vi "QMH_Tester_rev1.vi"() -> ()   [LabVIEW 2024]
doc: "Demonstrates the fundamentals of the Queued Message Handler design pattern in LabVIEW. A queued message handler, in its simplest form, is composed of two loops. The Event Handling Loop responds to user interface events by enqueuing \"messages\" on a message queue. These messages are dequeued in the Message Handling Loop. Note that the Message Handling Loop is also capable of sending messages to itself."
uses:
  Controls/Control_Stop.ctl
  Controls/Control_Unitherm Connect Disconnect Bool.ctl
  Controls/Control_M4X Connect Disconnect Bool.ctl
  Controls/Control_Fornax Connect Disconnect Bool.ctl
  Controls/Control_Unitherm Set Load Numeric.ctl
  Controls/Control_Unitherm Set Load Bool.ctl
  Controls/Control_Unitherm VISA Resource.ctl
  Controls/Control_Unitherm Clear Load Bool.ctl
  Controls/Control_PXI-7854R Connect Disconnect Bool.ctl
  Controls/Control_PXI-7854R 75kHz Bool.ctl
  Controls/Control_PXI-7854R uSec Off Numeric.ctl
  Controls/Control_PXI-7854R uSec On Numeric.ctl
  Controls/Control_PXI-7854R Resource.ctl
  Controls/Control_PXI-7854R Set Config Bool.ctl
  Controls/Control_PXI-7854R Set Config Enum.ctl
  Controls/Control_M4X Read Current Bool.ctl
  Controls/Control_Fornax Set Monopolar Command - Energy Channel ID Enum.ctl
  Controls/Control_Fornax Set Monopolar Command Bool.ctl
  Controls/Control_Fornax Set Monopolar Command - Cut Mode Enum.ctl
  Controls/Control_Fornax Set Monopolar Command - Coag Mode Enum.ctl
  Controls/Control_Fornax Set Monopolar Command - Cut Power Command Enum.ctl
  Controls/Control_Fornax Set Monopolar Command - Coag Power Command Enum.ctl
  Controls/Control_Fornax Set Monopolar Command - Serial Number String.ctl
  Program Files/National Instruments/LabVIEW 2024/examples/Design Patterns/Queued Message Handler/support/QMH Fundamentals - Message Cluster.ctl
  Controls/Control_Message Handling Cluster.ctl
  Controls/Control_M4X Connection.ctl
  Controls/Control_PXI-7854R FPGA Reference.ctl
  Controls/Control_Unitherm Connect Disconnect Cluster.ctl
  Controls/Control_PXI-7854R Connect Disconnect Cluster.ctl
  Controls/Control_Fornax Set Monopolar Command Cluster.ctl
  Controls/Control_PXI-7854R Set Config Cluster.ctl
  <vilib>/Utility/error.llb/Error Cluster From Error Code.vi
  <vilib>/rvi/errors/niLvFpgaAdjustHostInterfaceError.vi
  <vilib>/rvi/interface/nirviReadWriteControl/nirviReadWriteControl.xnode
  <vilib>/ErrorRing/Error Ring.xnode
  NiFpgaLv.dll
  <vilib>/rvi/interface/Simulation/niFpgaSimulationCallBeginRW.vi
  <vilib>/rvi/interface/nirviCloseFPGA/nirviCloseFPGA.xnode
  <vilib>/FPGAPlugInAG/Dynamic/niLvFpga_Close_Dynamic.vi
  <vilib>/userDefined/High Color/nirio_resource_hc.ctl
panel:
  in  "Serial Number":T1="T5G00443DX"
  in  "CoagPowerCommand":T2
  in  "CutPowerCommand":T3
  in  "CoagMode":T4
  in  "CutMode":T5
  in  "Fornax Set Monopolar Command":T6
  in  "EnergyChannelID":T7
  out "Data":waveform(dbl)[](graph)
  out "Array":T8(array[cluster])
  in  "Read Current":T9
  in  "7854 Config Enum":T10=enum."Off"
  in  "7854 Set Config":T11
  in  "resource name":T12="PXI1Slot6" caption="RIO Device"
  in  "uSec On":T13=7
  in  "uSec Off":T14=6
  in  "75kHz":T15=TRUE
  in  "7854 Connect/Disconnect":T16
  out "PXI-7854R Connected?":bool
  in  "Clear Load":T17
  in  "Unitherm Refnum in":T18="COM4"
  in  "Set Load":T19
  in  "Load (Ohms)":T20
  out "M4X Connected?":bool
  in  "Fornax Connect/Disconnect":T21
  in  "M4X Connect/Disconnect":T22
  in  "Unitherm Connect/Disconnect":T23
  out "Unitherm Connected?":bool
  out "Fornax Connected?":bool
  out "Display Message":string="\"Stop\" button pressed"
  in  "Fornax Action 1":bool
  in  "Stop":T24
  # "Unitherm"
  # "PXI-7854R"
  # "Fornax"
  # "M4X"
  # "Set Monopolar Command"
  # "Note: If you are creating a LabVIEW application based on the Queued Message Handler design pattern, create a Queued Message Handler project from the File > Create Project dialog."
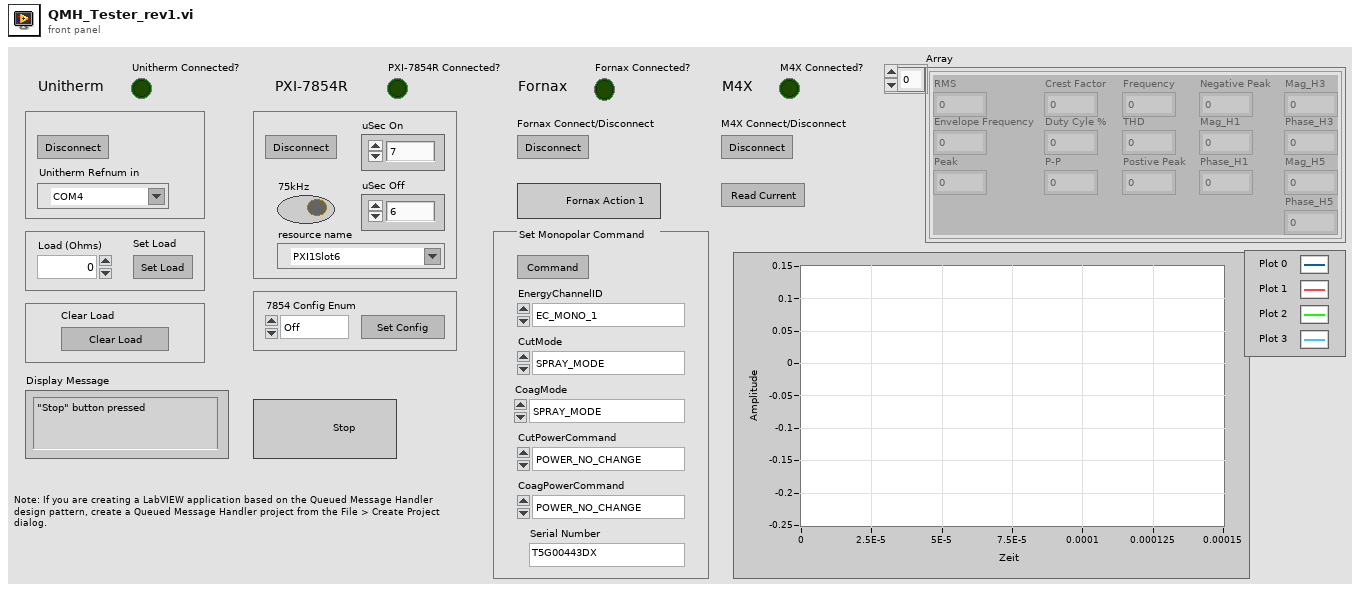
[diagram p1: front panel]
types:
  T1 = typedef "Control_Fornax Set Monopolar Command - Serial Number String.ctl" = string
  T2 = typedef "Control_Fornax Set Monopolar Command - Coag Power Command Enum.ctl" = enum16{"POWER_NO_CHANGE", "POWER_INCREASE", "POWER_DECREASE", "POWER_INCREASE_REPEAT", "POWER_DECREASE_REPEAT"}
  T3 = typedef "Control_Fornax Set Monopolar Command - Cut Power Command Enum.ctl" = enum16{"POWER_NO_CHANGE", "POWER_INCREASE", "POWER_DECREASE", "POWER_INCREASE_REPEAT", "POWER_DECREASE_REPEAT"}
  T4 = typedef "Control_Fornax Set Monopolar Command - Coag Mode Enum.ctl" = enum16{"SPRAY_MODE", "CUT_MODE", "BLEND_MODE", "FULGERATE_MODE", "BEPOLAR_MODE", "VESSEL_SEALING_MODE", "VALLEYLAB_MODE", "BIPOLAR_RESECTION_CUT_MODE", "BIPOLAR_RESECTION_COAG_MODE", "AUTOBIPOLAR_MODE", "VIPER_HLA", "SOFT_COAG_MODE", "NUM_ENERGY_MODES"}
  T5 = typedef "Control_Fornax Set Monopolar Command - Cut Mode Enum.ctl" = enum16{"SPRAY_MODE", "CUT_MODE", "BLEND_MODE", "FULGERATE_MODE", "BIPOLAR_MODE", "VESSEL_SEALING_MODE", "VALLEYLAB_MODE", "BIPOLAR_RESECTION_CUT_MODE", "BIPOLAR_RESECTION_COAG_MODE", "AUTOBIPOLAR_MODE", "VIPER_HLA", "SOFT_COAG_MODE", "NUM_ENERGY_MODES"}
  T6 = typedef "Control_Fornax Set Monopolar Command Bool.ctl" = bool
  T7 = typedef "Control_Fornax Set Monopolar Command - Energy Channel ID Enum.ctl" = enum16{"EC_MONO_1", "EC_BIPOLAR", "EC_MONO_2", "EC_ADVANCED", "NUM_ENERGY_CHANNELS", "EC_NOT_USED"}
  T8 = cluster{"RMS":dbl, "Envelope Frequency":dbl, "Peak":dbl, "Crest Factor":dbl, "Duty Cyle %":dbl, "P-P":dbl, "Frequency":dbl, "THD":dbl, "Postive Peak":dbl, "Negative Peak":dbl, "Mag_H1":dbl, "Phase_H1":dbl, "Mag_H3":dbl, "Phase_H3":dbl, "Mag_H5":dbl, "Phase_H5":dbl}[]
  T9 = typedef "Control_M4X Read Current Bool.ctl" = bool
  T10 = typedef "Control_PXI-7854R Set Config Enum.ctl" = enum16{"Mono 1", "Mono 2", "BiPolar", "LigaSure", "Off"}
  T11 = typedef "Control_PXI-7854R Set Config Bool.ctl" = bool
  T12 = typedef "Control_PXI-7854R Resource.ctl" = tag
  T13 = typedef "Control_PXI-7854R uSec On Numeric.ctl" = u16
  T14 = typedef "Control_PXI-7854R uSec Off Numeric.ctl" = u16
  T15 = typedef "Control_PXI-7854R 75kHz Bool.ctl" = bool
  T16 = typedef "Control_PXI-7854R Connect Disconnect Bool.ctl" = bool
  T17 = typedef "Control_Unitherm Clear Load Bool.ctl" = bool
  T18 = typedef "Control_Unitherm VISA Resource.ctl" = refnum<visa-resource-name>
  T19 = typedef "Control_Unitherm Set Load Bool.ctl" = bool
  T20 = typedef "Control_Unitherm Set Load Numeric.ctl" = i32
  T21 = typedef "Control_Fornax Connect Disconnect Bool.ctl" = bool
  T22 = typedef "Control_M4X Connect Disconnect Bool.ctl" = bool
  T23 = typedef "Control_Unitherm Connect Disconnect Bool.ctl" = bool
  T24 = typedef "Control_Stop.ctl" = bool
  T25 = typedef "Control_Message Handling Cluster.ctl" = cluster{"Fornax Connected?":refnum<vi>, "Unitherm Connected?":refnum<vi>, "M4X Connected?":refnum<vi>, "Unitherm Connect/Disconnect":refnum<vi>, "Fornax Connection":refnum<k5>, "UNITHERM Connection":refnum<visa-resource-name>, "M4X Connection":T26, "PXI-7854R FPGA Reference":T27, "PXI-7854R Connected?":refnum<vi>, "Fornax Connect/Disconnect":refnum<vi>, "7854 Connect/Disconnect":refnum<vi>, "M4X Connect/Disconnect":refnum<vi>}
  T26 = typedef "Control_M4X Connection.ctl" = u32
  T27 = typedef "Control_PXI-7854R FPGA Reference.ctl" = refnum<k20>
  T28 = typedef "QMH Fundamentals - Message Cluster.ctl" = cluster{"Message":string, "Message Data":variant}
  T29 = typedef "Control_PXI-7854R Set Config Cluster.ctl" = cluster{"7854 Config Enum":T10, "7854 Set Config":T11}
  T30 = typedef "nirio_resource_hc.ctl" = tag
  T31 = typedef "Control_Unitherm Connect Disconnect Cluster.ctl" = cluster{"Unitherm Connect/Disconnect":T23, "Unitherm Refnum in":T18}
  T32 = typedef "Control_PXI-7854R Connect Disconnect Cluster.ctl" = cluster{"PXI-7854R Resource":T12, "75kHz":T15, "uSec Off":T14, "uSec On":T13, "7854 Connect/Disconnect":T16}
  T33 = enum16{"EXTERNAL_COMM_COMMAND_INVALID", "EXTERNAL_COMM_COMMAND_PAIR_VLEX", "EXTERNAL_COMM_COMMAND_PAIR_FORNAX", "EXTERNAL_COMM_COMMAND_PAIR_INTEGRATION_TESTOR", "EXTERNAL_COMM_COMMAND_ENABLE_DFA", "EXTERNAL_COMM_COMMAND_ENABLE_DFT", "EXTERNAL_COMM_COMMAND_ENABLE_VIPER", "EXTERNAL_COMM_COMMAND_AUTO_ETHERNET_ON", "EXTERNAL_COMM_COMMAND_AUTO_ETHERNET_OFF", "EXTERNAL_COMM_COMMAND_STREAM_RFDATA_ON", "EXTERNAL_COMM_COMMAND_STREAM_RFDATA_OFF", "EXTERNAL_COMM_COMMAND_STREAM_ISOFIRM_ON", "EXTERNAL_COMM_COMMAND_STREAM_ISOFIRM_OFF", "EXTERNAL_COMM_COMMAND_STREAM_RFID_ON", "EXTERNAL_COMM_COMMAND_STREAM_RFID_OFF", "EXTERNAL_COMM_COMMAND_AUTO_ETHERNET_ONCE"}
  T34 = typedef "Control_Fornax Set Monopolar Command Cluster.ctl" = cluster{"Serial Number":T1, "EnergyChannelID":T7, "CutMode":T5, "CoagMode":T4, "CutPowerCommand":T3, "CoagPowerCommand":T2, "Fornax Set Monopolar Command":T6}
  T35 = cluster{"RMS":dbl, "Envelope Frequency":dbl, "Peak":dbl, "Crest Factor":dbl, "Duty Cyle %":dbl, "P-P":dbl, "Frequency":dbl, "THD":dbl, "Postive Peak":dbl, "Negative Peak":dbl, "Mag_H1":dbl, "Phase_H1":dbl, "Mag_H3":dbl, "Phase_H3":dbl, "Mag_H5":dbl, "Phase_H5":dbl}
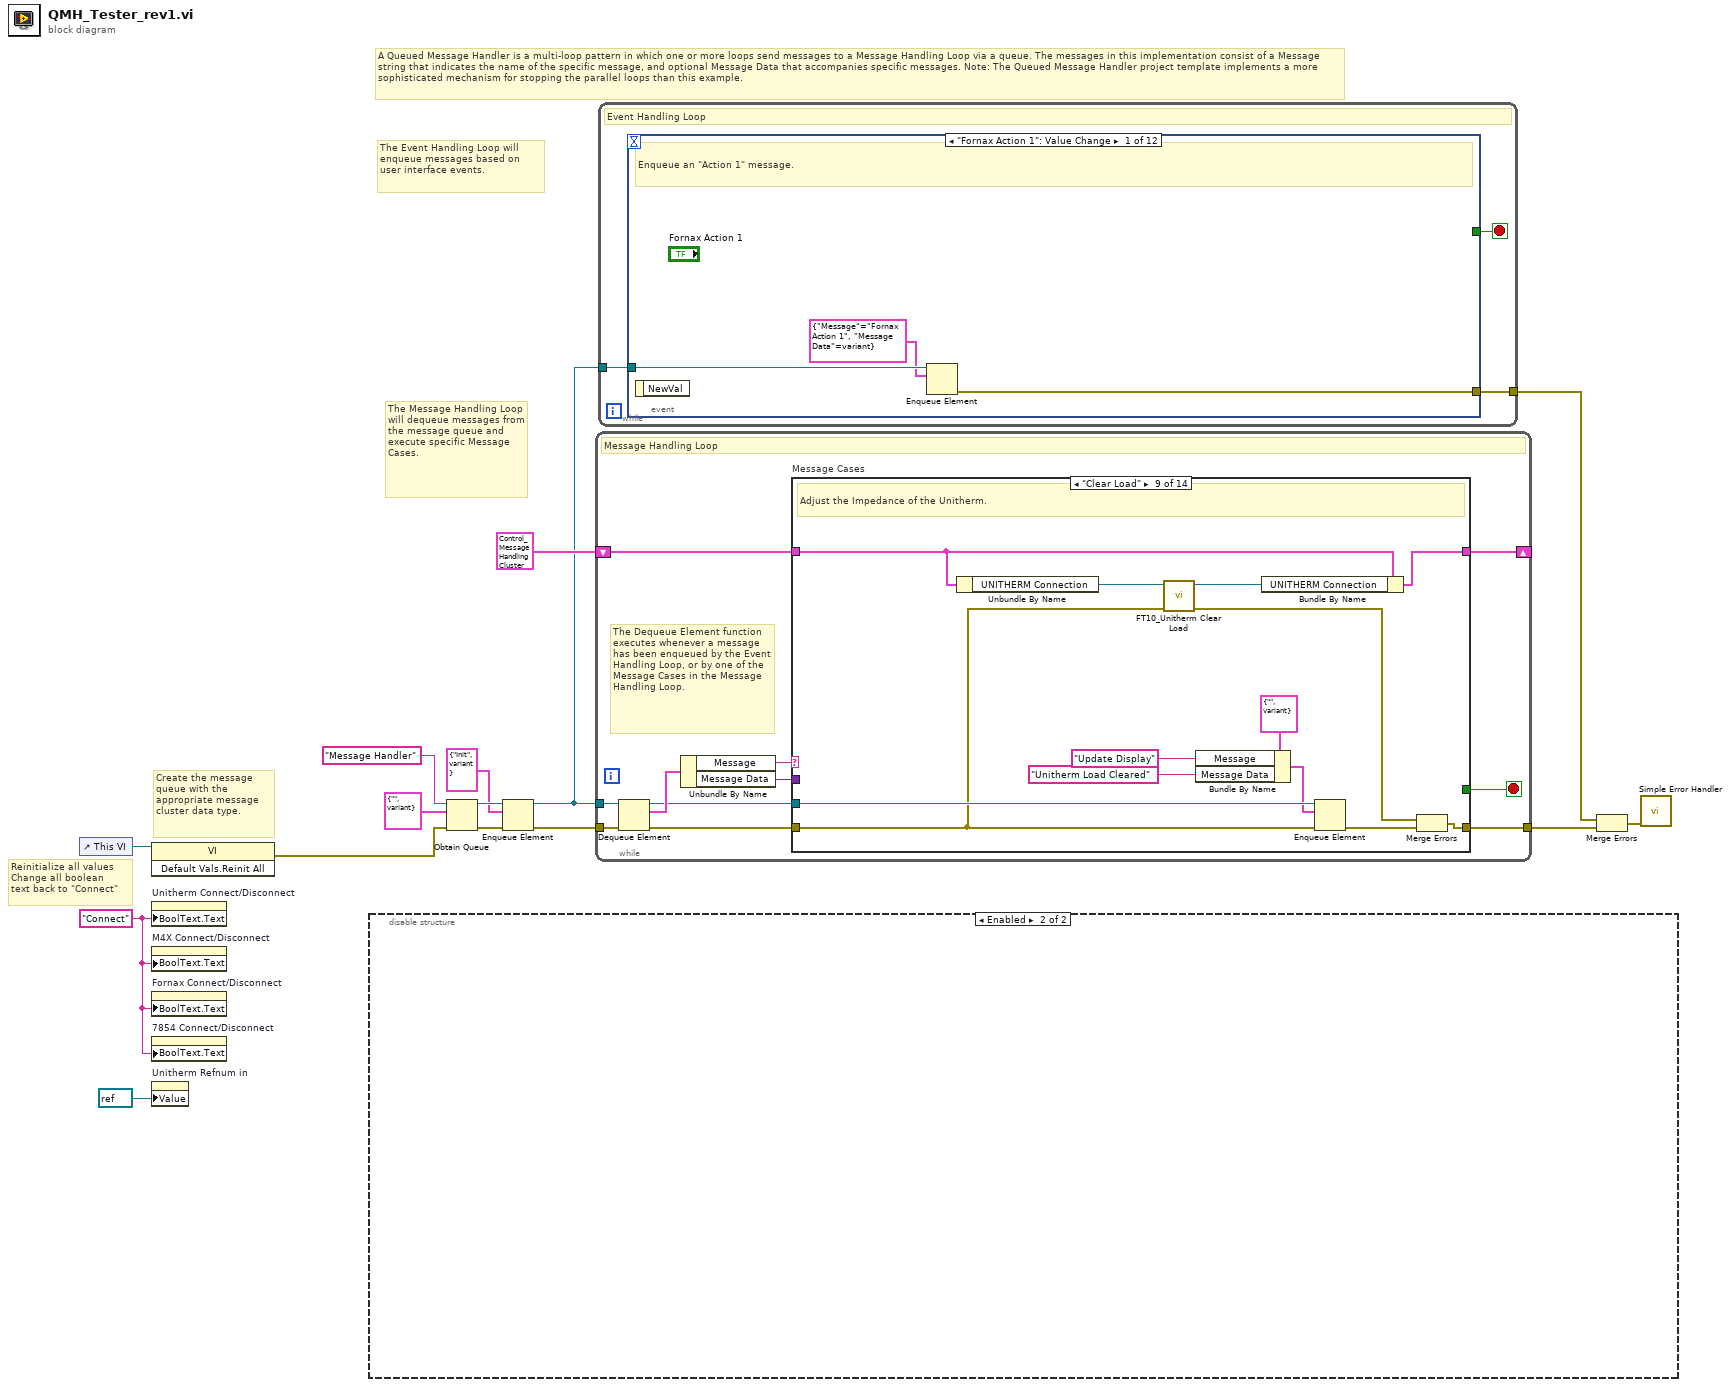
[diagram p0: block diagram]
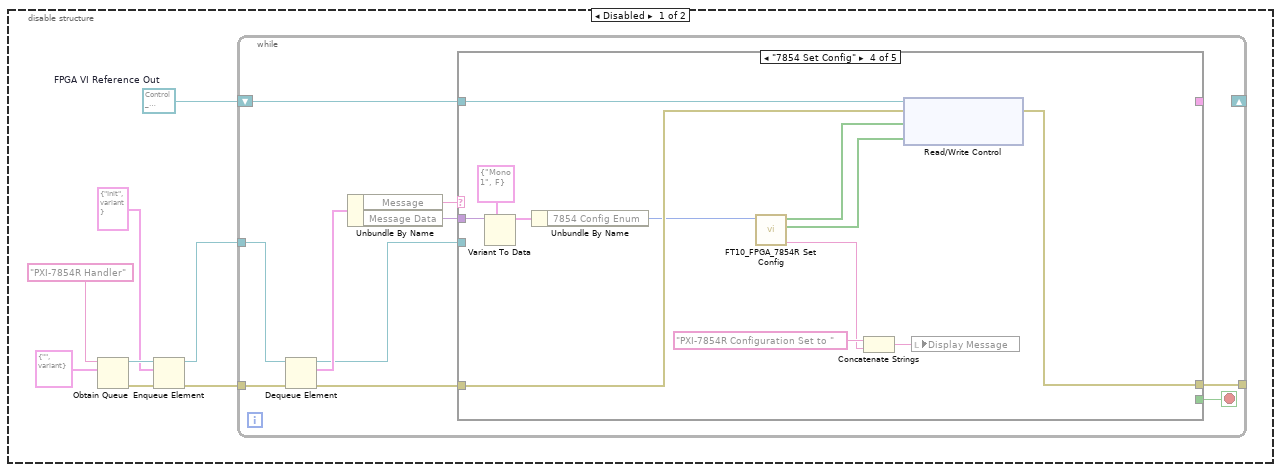
[diagram p2: hidden frame]
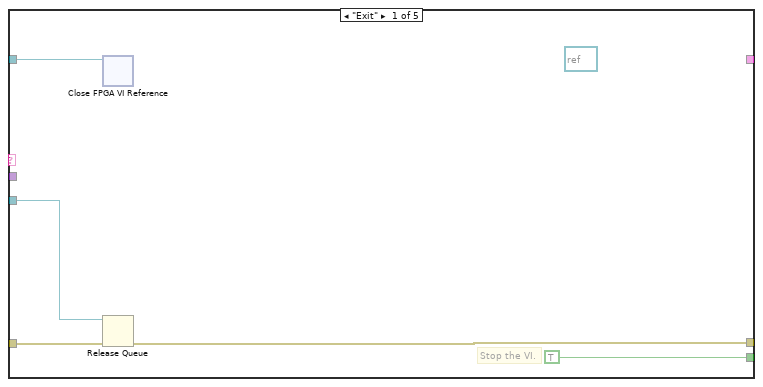
[diagram p3: hidden frame]
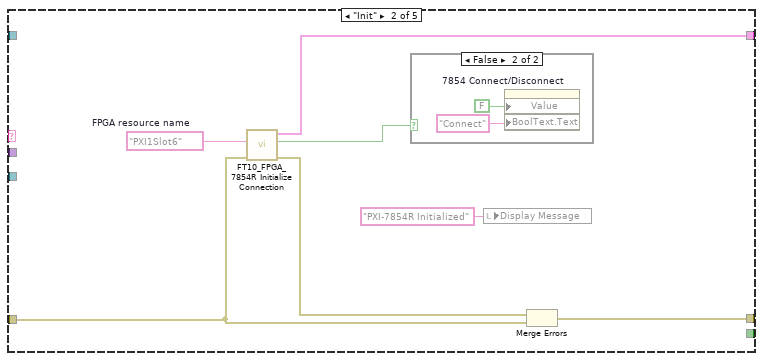
[diagram p4: hidden frame]
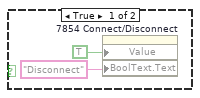
[diagram p5: hidden frame]
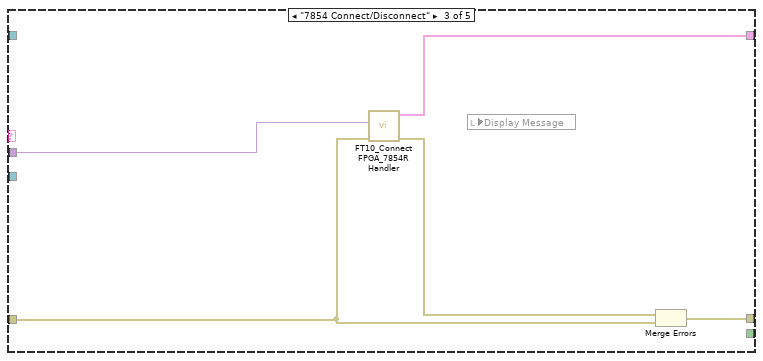
[diagram p6: hidden frame]
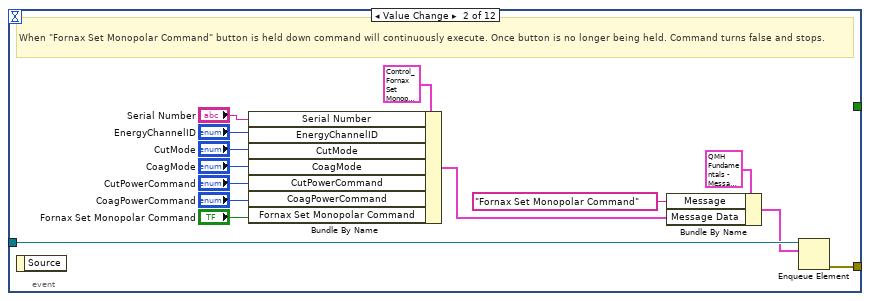
[diagram p8: hidden frame]
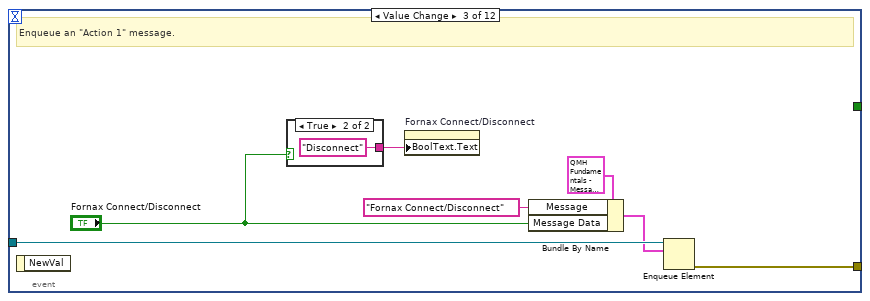
[diagram p9: hidden frame]
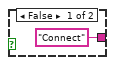
[diagram p10: hidden frame]
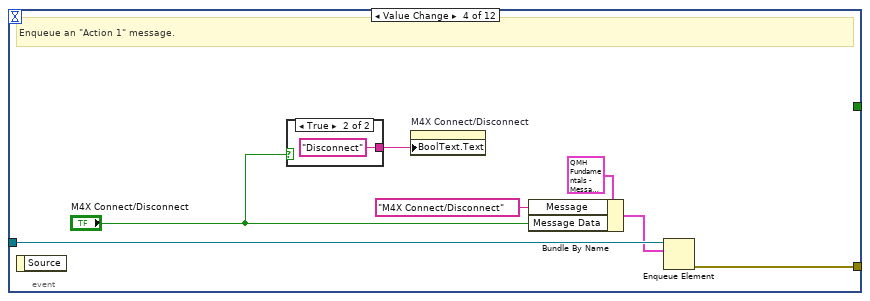
[diagram p11: hidden frame]
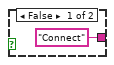
[diagram p12: hidden frame]
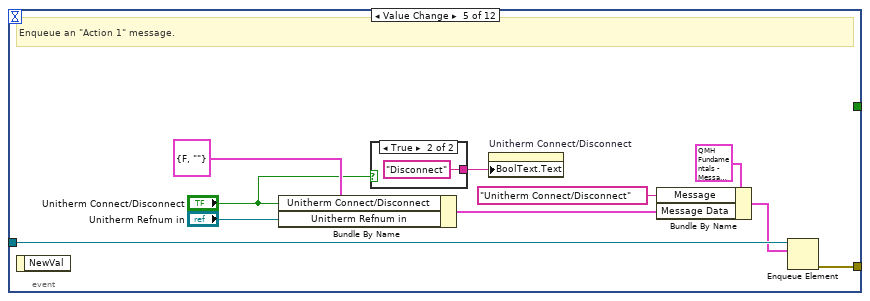
[diagram p13: hidden frame]
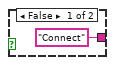
[diagram p14: hidden frame]
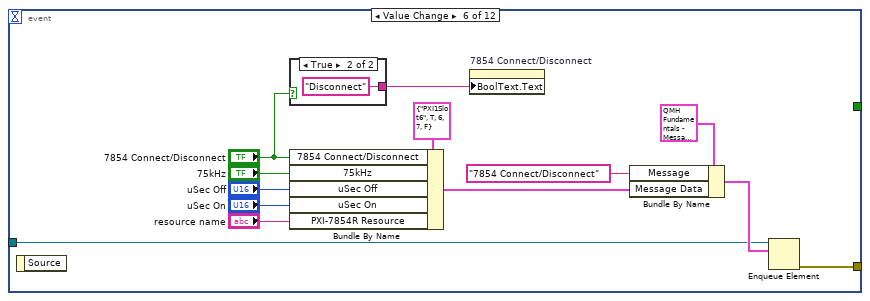
[diagram p15: hidden frame]
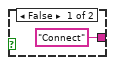
[diagram p16: hidden frame]
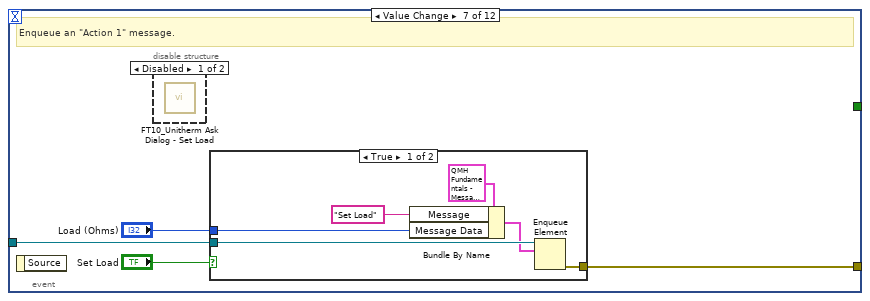
[diagram p17: hidden frame]
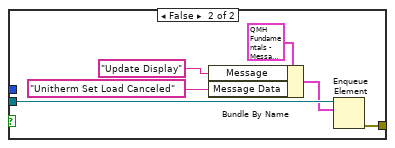
[diagram p19: hidden frame]
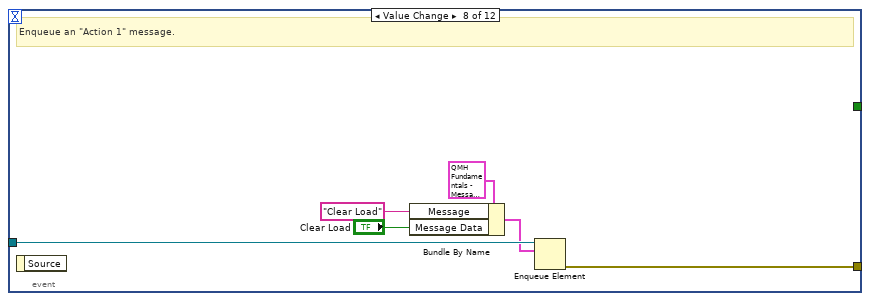
[diagram p20: hidden frame]
diagram:
  w1 = "Connect" ("Boolean Text.Text")
  # "Reinitialize all values\nChange all boolean\ntext back to \"Connect\""
  # "Create the message queue with the appropriate message cluster data type."
  # "A Queued Message Handler is a multi-loop pattern in which one or more loops send messages to a Message Handling Loop via a queue. The messages in this implementation consist of a Message string that indicates the name of the specific message, and optional Message Data that accompanies specific messages. Note: The Queued Message Handler project template implements a more sophisticated mechanism for stopping the parallel loops than this example."
  # "The Message Handling Loop will dequeue messages from the message queue and execute specific Message Cases."
  # "The Event Handling Loop will enqueue messages based on user interface events."
  n1 = control-ref of="This VI"() -> (w6:refnum<vi>)
  n2 = invoke class="VI" method="Default Vals.Reinit All"(reference=w6) -> (error out=w5:errorcluster)  [unwired: 2 in, 2 out]
  n3 = property on="Unitherm Connect/Disconnect" class="Bool (strict)"("BoolText.Text"=w1) -> ()  [unwired: 2 in, 2 out]
  n4 = property on="M4X Connect/Disconnect" class="Bool (strict)"("BoolText.Text"=w1) -> ()  [unwired: 2 in, 2 out]
  n5 = property on="Fornax Connect/Disconnect" class="Bool (strict)"("BoolText.Text"=w1) -> ()  [unwired: 2 in, 2 out]
  n6 = property on="7854 Connect/Disconnect" class="Bool (strict)"("BoolText.Text"=w1) -> ()  [unwired: 2 in, 2 out]
  n7 = property on="Unitherm Refnum in" class="VISAName (strict)"("Value"=refnum<visa-resource-name> refnum ("Unitherm Refnum in")) -> ()  [unwired: 2 in, 2 out]
  n8 = disable-structure shown="Enabled" {
    frame Disabled {
      w19 = T27 refnum  # FPGA VI Reference Out
      n9 = Obtain Queue(name (unnamed)="PXI-7854R Handler", element data type=T28 {"Message"="", "Message Data"=variant} ("Message Cluster")) -> (queue out=w23:refnum<queue>, error out=w20:errorcluster)  [unwired: 3 in, 1 out]
      n10 = Enqueue Element(queue=w23, element=T28 {"Message"="Init", "Message Data"=variant}, error in (no error)=w20) -> (queue out=w18:refnum<queue>, error out=w17:errorcluster)  [unwired: 1 in, 1 out]
      n11 = while {
        tunnel: w18 -> [w33]
        tunnel: w17 -> [w32]
        shift-right: _ -> [_]
        shift-left: w19 -> [w25]
        tunnel: [w27] -> w16
        stop <- w30 stop-if-true
        n12 = Dequeue Element(queue=w33, error in (no error)=w32) -> (queue out=w29:refnum<queue>, element=w34:T28, error out=w28:errorcluster)  [unwired: 1 in, 1 out]
        n13 = Unbundle By Name(w34) -> ("Message"=w31:string, "Message Data"=w26:variant)
        n14 = case shown="\"7854 Set Config\"" w31 {
          tunnel: [TRUE _ _ _ _] -> w30
          tunnel: w29 -> [w38 _ _ _ _]
          tunnel: w28 -> [w37 w41 w53 w61 w68]
          tunnel: [_ w40 w51 _ _] -> _
          tunnel: w25 -> [w35 _ _ w64 _]
          tunnel: [w36 w45 w55 w60 w68] -> w27
          tunnel: w26 -> [_ _ w54 w66 _]
          frame "Exit" {
            (unwired) refnum<k20> refnum ("FPGA VI Reference Out")
            # "Stop the VI."
            n15 = xnode "Close FPGA VI Reference"("FPGA VI Reference In"=w35) -> ()  [unwired: 1 in, 1 out]
            n16 = Release Queue(queue=w38, error in (no error)=w37) -> (error out=w36:errorcluster)  [unwired: 1 in, 2 out]
          }
          frame "Init" {
            w46 = T30 "PXI1Slot6"  # FPGA resource name
            n17 = call "FT10_FPGA_7854R Initialize Connection.vi"("error in"=w41, "FPGA resource name"=w46) -> ("error out"=w44:errorcluster, "PXI-7854R Connected?"=w42:bool, "Message Handling Cluster out"=w40:T25)  [unwired: 7 in]
            n18 = case shown="False" w42 {
              frame True {
                n19 = property on="7854 Connect/Disconnect" class="Bool (strict)"("Value"=TRUE ("7854 Connect/Disconnect"), "BoolText.Text"="Disconnect" ("Boolean Text.Text")) -> ()  [unwired: 2 in, 2 out]
              }
              frame False {
                n20 = property on="7854 Connect/Disconnect" class="Bool (strict)"("Value"=FALSE ("7854 Connect/Disconnect"), "BoolText.Text"="Connect" ("Boolean Text.Text")) -> ()  [unwired: 2 in, 2 out]
              }
            }
            n21 = local write "Display Message"("PXI-7854R Initialized" ("Display Message")) -> ()
            n22 = Merge Errors(w44, w41) -> (w45:errorcluster)
          }
          frame "7854 Connect/Disconnect" {
            n23 = call "FT10_Connect FPGA_7854R Handler.vi"("error in"=w53, "Message Data"=w54) -> ("error out"=w52:errorcluster, "Message Handling Cluster out"=w51:T25)  [unwired: 7 in, 1 out]
            n24 = local read "Display Message"() -> ()  [unwired: 1 in]
            n25 = Merge Errors(w52, w53) -> (w55:errorcluster)
          }
          frame "7854 Set Config" {
            n26 = Variant To Data(type=T29 {"7854 Config Enum"=enum."Mono 1", "7854 Set Config"=FALSE}, Variant=w66) -> (data=w65:T29)  [unwired: 1 in, 1 out]
            n27 = Unbundle By Name(w65) -> ("7854 Config Enum"=w57:T10)
            n28 = call "FT10_FPGA_7854R Set Config.vi"("7854 Config Enum"=w57) -> ("Config string"=w56:string, "Conn2/DIO_8_15 In"=w62:bool[], "Conn2/DIO_0_7 In"=w63:bool[])  [unwired: 8 in]
            n29 = Concatenate Strings("PXI-7854R Configuration Set to " ("Display Message"), w56) -> (w58:string)
            n30 = xnode "Read/Write Control"("FPGA VI Reference In"=w64, "error in"=w61, "Conn2/DIO_0_7 In"=w63, "Conn2/DIO_8_15 In"=w62) -> ("error out"=w60:errorcluster)  [unwired: 1 out]
            n31 = local write "Display Message"(w58) -> ()
          }
          frame Default {
          }
        }
      }
    }
    frame Enabled {
    }
  }
  n32 = Obtain Queue(name (unnamed)="Message Handler", element data type=T28 {"Message"="", "Message Data"=variant} ("Message Cluster"), error in (no error)=w5) -> (queue out=w11:refnum<queue>, error out=w12:errorcluster)  [unwired: 2 in, 1 out]
  n33 = Enqueue Element(queue=w11, element=T28 {"Message"="Init", "Message Data"=variant}, error in (no error)=w12) -> (queue out=w2:refnum<queue>, error out=w10:errorcluster)  [unwired: 1 in, 1 out]
  n34 = while {
    tunnel: w2 -> [w76]
    tunnel: w10 -> [w77]
    tunnel: [w78] -> w15
    shift-right: [w69] -> _
    shift-left: T25 {"Fornax Connected?"=refnum, "Unitherm Connected?"=refnum, "M4X Connected?"=refnum, "Unitherm Connect/Disconnect"=refnum, "Fornax Connection"=refnum, "UNITHERM Connection"="", "M4X Connection"=0, "PXI-7854R FPGA Reference"=refnum, "PXI-7854R Connected?"=refnum, "Fornax Connect/Disconnect"=refnum, "7854 Connect/Disconnect"=refnum, "M4X Connect/Disconnect"=refnum} -> [w70]
    stop <- w79 stop-if-true
    # "The Dequeue Element function executes whenever a message has been enqueued by the Event Handling Loop, or by one of the Message Cases in the Message Handling Loop."
    # "Message Handling Loop"
    n35 = Dequeue Element(queue=w76, error in (no error)=w77) -> (queue out=w74:refnum<queue>, element=w75:T28, error out=w73:errorcluster)  [unwired: 1 in, 1 out]
    n36 = Unbundle By Name(w75) -> ("Message"=w72:string, "Message Data"=w71:variant)
    n37 = case "Message Cases" shown="\"Clear Load\"" w72 {
      selector: w72 -> [_ _ _ _ _ _ _ _ _ _ _ _ _ w336]
      tunnel: w74 -> [w98 w115 w134 w163 w182 w204 w213 w252 w265 w289 w293 _ w332 _]
      tunnel: w73 -> [w91 w114 w125 w154 w173 w190 w210 w238 w254 w280 w296 w317 w322 w335]
      tunnel: [w99 w116 w135 w164 w183 w193 w212 w244 w258 w282 w297 w314 w324 w335] -> w78
      tunnel: [_ _ _ _ _ _ _ _ _ _ _ _ TRUE _] -> w79
      tunnel: w71 -> [_ w109 w132 w153 w174 _ w211 w242 _ _ w305 w316 _ _]
      tunnel: w70 -> [w97 w120 w127 w158 w176 w195 w206 w245 w259 w283 w308 w312 w326 w333]
      tunnel: [w92 w113 w126 w157 w175 w196 w205 w246 w260 w284 w307 w312 w325 w333] -> w69
      frame "Init" {
        # "Initialize - Create reference for connection indicators. Connect to Fornax, M4X, and Unitherm."
        n38 = control-ref of="Fornax Connected?"() -> (w96:refnum<vi>)
        n39 = control-ref of="Unitherm Connected?"() -> (w95:refnum<vi>)
        n40 = control-ref of="M4X Connected?"() -> (w94:refnum<vi>)
        n41 = control-ref of="PXI-7854R Connected?"() -> (w85:refnum<vi>)
        n42 = control-ref of="Unitherm Connect/Disconnect"() -> (w83:refnum<vi>)
        n43 = control-ref of="Fornax Connect/Disconnect"() -> (w82:refnum<vi>)
        n44 = control-ref of="7854 Connect/Disconnect"() -> (w81:refnum<vi>)
        n45 = control-ref of="M4X Connect/Disconnect"() -> (w80:refnum<vi>)
        n46 = Bundle By Name(cluster=w97, "Fornax Connected?"=w96, "Unitherm Connected?"=w95, "M4X Connected?"=w94, "PXI-7854R Connected?"=w85, "UNITHERM Connection"=refnum<visa-resource-name> "COM4", "Unitherm Connect/Disconnect"=w83, "Fornax Connect/Disconnect"=w82, "7854 Connect/Disconnect"=w81, "M4X Connect/Disconnect"=w80) -> (w93:T25)
        n47 = Bundle By Name(cluster=T28 {"Message"="", "Message Data"=variant} ("Message Cluster"), "Message"="Update Display", "Message Data"="Initialize Complete" ("L10n_Action 1 Pressed")) -> (w102:T28)
        n48 = call "FT10_Connect Hardware.vi"("Message Handling Cluster in"=w93, "error in (no error)"=w91) -> ("Message Handling Cluster out"=w92:T25, "Fornax Connected?"=→"Fornax Connected?":bool, "Unitherm Connected?"=→"Unitherm Connected?":bool, "M4X Connected?"=→"M4X Connected?":bool, "PXI-7854R Connected?"=→"PXI-7854R Connected?":bool, "error out"=w90:errorcluster)  [unwired: 8 in]
        n49 = Enqueue Element(queue=w98, element=w102, error in (no error)=w91) -> (error out=w100:errorcluster)  [unwired: 1 in, 2 out]
        n50 = Merge Errors(w90, w100) -> (w99:errorcluster)
      }
      frame "Fornax Connect/Disconnect" {
        # "Connect or disconnect from Fornax."
        n51 = Variant To Data(type=TRUE, Variant=w109) -> (data=w106:bool)  [unwired: 1 in, 1 out]
        n52 = case shown="True" w106 {
          tunnel: ["Fornax Disconnect" ("L10n_Action 1 Pressed") "Fornax Connect" ("L10n_Action 1 Pressed")] -> w105
          frame False {
          }
          frame True {
          }
        }
        n53 = call "FT10_Connect Fornax Handler.vi"("error in (no error)"=w114, "Message Data"=w109, "Message Handling Cluster in"=w120) -> ("error out"=w111:errorcluster, "Fornax Connected?"=w110:bool, "Message Handling Cluster out"=w113:T25)  [unwired: 6 in]
        n54 = Bundle By Name(cluster=T28 {"Message"="", "Message Data"=variant} ("Message Cluster"), "Message Data"=w105, "Message"="Update Display") -> (w118:T28)
        n55 = Enqueue Element(queue=w115, element=w118, error in (no error)=w114) -> (error out=w117:errorcluster)  [unwired: 1 in, 2 out]
        n56 = Unbundle By Name(w113) -> ("Fornax Connected?"=w112:refnum<vi>)
        n57 = property class="Bool (strict)"(reference=w112, "Value"=w110) -> ()  [unwired: 1 in, 2 out]
        n58 = Merge Errors(w111, w117) -> (w116:errorcluster)
      }
      frame "M4X Connect/Disconnect" {
        # "Connect or disconnect from M4X."
        n59 = Variant To Data(type=TRUE, Variant=w132) -> (data=w129:bool)  [unwired: 1 in, 1 out]
        n60 = case shown="True" w129 {
          tunnel: ["M4X Disconnect" ("L10n_Action 1 Pressed") "M4X Connect" ("L10n_Action 1 Pressed")] -> w128
          tunnel: w127 -> [w141 w147]
          tunnel: [w141 w146] -> w126
          tunnel: w125 -> [w140 w145]
          tunnel: [w140 w144] -> w124
          tunnel: [FALSE ("M4X Connected?") w143] -> w123
          frame False {
          }
          frame True {
            n61 = call "FT10_Connect M4X.vi"("error in (no error)"=w145, "reset device"=TRUE, "Board #"=u32 0, "Message Handling Cluster in"=w147) -> ("error out"=w144:errorcluster, "M4X Connected?"=w143:bool, "Message Handling Cluster out"=w146:T25)  [unwired: 4 in, 1 out]
          }
        }
        n62 = Bundle By Name(cluster=T28 {"Message"="", "Message Data"=variant} ("Message Cluster"), "Message Data"=w128, "Message"="Update Display") -> (w137:T28)
        n63 = Enqueue Element(queue=w134, element=w137, error in (no error)=w125) -> (error out=w136:errorcluster)  [unwired: 1 in, 2 out]
        n64 = Unbundle By Name(w126) -> ("M4X Connected?"=w133:refnum<vi>)
        n65 = property class="Bool (strict)"(reference=w133, "Value"=w123) -> ()  [unwired: 1 in, 2 out]
        n66 = Merge Errors(w124, w136) -> (w135:errorcluster)
      }
      frame "Unitherm Connect/Disconnect" {
        # "Connect or disconnect from Unitherm."
        n67 = Variant To Data(type=T31 {"Unitherm Connect/Disconnect"=FALSE, "Unitherm Refnum in"=""}, Variant=w153) -> (data=w160:T31)  [unwired: 1 in, 1 out]
        n68 = Unbundle By Name(w160) -> ("Unitherm Connect/Disconnect"=w151:T23)
        n69 = call "FT10_Connect Unitherm Handler.vi"("error in (no error)"=w154, "Message Data"=w153, "Message Handling Cluster in"=w158) -> ("error out"=w155:errorcluster, "Unitherm Connected?"=w156:bool, "Message Handling Cluster out"=w157:T25)  [unwired: 6 in]
        n70 = case shown="False" w151 {
          tunnel: ["Unitherm Disconnect" ("L10n_Action 1 Pressed") "Unitherm Connect" ("L10n_Action 1 Pressed")] -> w159
          frame False {
          }
          frame True {
          }
        }
        n71 = Unbundle By Name(w157) -> ("Unitherm Connected?"=w162:refnum<vi>)
        n72 = Bundle By Name(cluster=T28 {"Message"="", "Message Data"=variant} ("Message Cluster"), "Message Data"=w159, "Message"="Update Display") -> (w166:T28)
        n73 = Enqueue Element(queue=w163, element=w166, error in (no error)=w154) -> (error out=w165:errorcluster)  [unwired: 1 in, 2 out]
        n74 = property class="Bool (strict)"(reference=w162, "Value"=w156) -> ()  [unwired: 1 in, 2 out]
        n75 = Merge Errors(w155, w165) -> (w164:errorcluster)
      }
      frame "7854 Connect/Disconnect" {
        # "Connect or disconnect from Unitherm."
        n76 = Variant To Data(type=T32 {"PXI-7854R Resource"="PXI1Slot6", "75kHz"=TRUE, "uSec Off"=6, "uSec On"=7, "7854 Connect/Disconnect"=FALSE}, Variant=w174) -> (data=w179:T32)  [unwired: 1 in, 1 out]
        n77 = Unbundle By Name(w179) -> ("7854 Connect/Disconnect"=w177:T16)
        n78 = case shown="False" w177 {
          tunnel: ["PXI-7854R Disconnected" ("L10n_Action 1 Pressed") "PXI-7854R Connected" ("L10n_Action 1 Pressed")] -> w178
          frame False {
          }
          frame True {
          }
        }
        n79 = call "FT10_Connect FPGA_7854R Handler.vi"("error in"=w173, "Message Data"=w174, "Message Handling Cluster in"=w176) -> ("error out"=w172:errorcluster, "PXI-7854R Connected?"=w171:bool, "Message Handling Cluster out"=w175:T25)  [unwired: 6 in]
        n80 = Unbundle By Name(w175) -> ("PXI-7854R Connected?"=w181:refnum<vi>)
        n81 = Bundle By Name(cluster=T28 {"Message"="", "Message Data"=variant} ("Message Cluster"), "Message Data"=w178, "Message"="Update Display") -> (w185:T28)
        n82 = Enqueue Element(queue=w182, element=w185, error in (no error)=w173) -> (error out=w184:errorcluster)  [unwired: 1 in, 2 out]
        n83 = property class="Bool (strict)"(reference=w181, "Value"=w171) -> ()  [unwired: 1 in, 2 out]
        n84 = Merge Errors(w172, w184) -> (w183:errorcluster)
      }
      frame "Fornax Action 1" {
        # "Action 1 - Send an \"Update Display\" message indicating which button was pressed. Note that a string is sent as the Message Data along with the \"Update Display\" message."
        n85 = Unbundle By Name(w195) -> ("Fornax Connection"=w198:refnum<k5>)
        n86 = call "FT10_Fornax Command.vi"("ExternalCommCommand"=T33."EXTERNAL_COMM_COMMAND_ENABLE_DFT") -> ("JSON Message"=w192:string)  [unwired: 10 in]
        n87 = Bundle By Name(cluster=T28 {"Message"="", "Message Data"=variant} ("Message Cluster"), "Message"="Update Display", "Message Data"="Fornax Action 1 button pressed" ("L10n_Action 1 Pressed")) -> (w200:T28)
        n88 = TCP Write(connection ID=w198, data in=w192, error in (no error)=w190, 9:100 ("timeout ms (25000)")) -> (connection ID out=w197:refnum<k5>, error out=w189:errorcluster)  [unwired: 1 out]
        n89 = Bundle By Name(cluster=w195, "Fornax Connection"=w197) -> (w196:T25)
        n90 = Enqueue Element(queue=w204, element=w200, error in (no error)=w190) -> (error out=w203:errorcluster)  [unwired: 1 in, 2 out]
        n91 = Merge Errors(w189, w203) -> (w193:errorcluster)
      }
      frame "Fornax Set Monopolar Command" {
        # "When \"Fornax Set Monopolar Command\" button is held down command will continuously execute. Once button is no longer being held. Command turns false and stops."
        n92 = Variant To Data(type=T34 {"Serial Number"="CAMM_INTERNAL_GENERIC", "EnergyChannelID"=enum."EC_MONO_1", "CutMode"=enum."SPRAY_MODE", "CoagMode"=enum."SPRAY_MODE", "CutPowerCommand"=enum."POWER_NO_CHANGE", "CoagPowerCommand"=enum."POWER_NO_CHANGE", "Fornax Set Monopolar Command"=FALSE}, Variant=w211) -> (data=w207:T34)  [unwired: 1 in, 1 out]
        n93 = Unbundle By Name(w207) -> ("Fornax Set Monopolar Command"=w208:T6)
        n94 = case shown="True" w208 {
          tunnel: w213 -> [w217 w233]
          tunnel: [w215 w232] -> w212
          tunnel: w210 -> [w216 w227]
          tunnel: w207 -> [w218 _]
          tunnel: w206 -> [w220 w226]
          tunnel: [w219 w226] -> w205
          frame True {
            n95 = call "FT10_Fornax Send MonopolarCommand.vi"("error in"=w216, "Set Monopolar Command Cluster in"=w218, "Message Handling Cluster in"=w220) -> ("error out"=w214:errorcluster, "Message Handling Cluster out"=w219:T25)  [unwired: 6 in, 1 out]
            n96 = Bundle By Name(cluster=T28 {"Message"="", "Message Data"=variant} ("Message Cluster"), "Message"="Update Display", "Message Data"="Fornax Command button pressed ON" ("L10n_Action 1 Pressed")) -> (w222:T28)
            n97 = Enqueue Element(queue=w217, element=w222, error in (no error)=w216) -> (error out=w225:errorcluster)  [unwired: 1 in, 2 out]
            n98 = Merge Errors(w214, w225) -> (w215:errorcluster)
          }
          frame False {
            n99 = Bundle By Name(cluster=T28 {"Message"="", "Message Data"=variant} ("Message Cluster"), "Message"="Update Display", "Message Data"="Fornax Command button pressed OFF" ("L10n_Action 1 Pressed")) -> (w229:T28)
            n100 = Enqueue Element(queue=w233, element=w229, error in (no error)=w227) -> (error out=w232:errorcluster)  [unwired: 1 in, 2 out]
          }
        }
      }
      frame "Set Load" {
        # "Adjust the Impedance of the Unitherm."
        n101 = Variant To Data(type=0 ("Load (Ohms)"), Variant=w242) -> (data=w237:i32)  [unwired: 1 in, 1 out]
        n102 = Number To Decimal String(number=w237) -> (decimal integer string=w235:string)  [unwired: 1 in]
        n103 = Unbundle By Name(w245) -> ("UNITHERM Connection"=w241:refnum<visa-resource-name>)
        n104 = Concatenate Strings("Unitherm Load set to " ("L10n_Action 1 Pressed"), w235, " Ohms" ("string")) -> (w236:string)
        n105 = call "FT10_Unitherm Set Load.vi"("error in (no error)"=w238, "Load Impedance"=w237, "VISA Refnum in"=w241) -> ("error out"=w239:errorcluster, "VISA Refnum out"=w240:refnum<visa-resource-name>)  [unwired: 7 in]
        n106 = Bundle By Name(cluster=T28 {"Message"="", "Message Data"=variant} ("Message Cluster"), "Message"="Update Display", "Message Data"=w236) -> (w248:T28)
        n107 = Bundle By Name(cluster=w245, "UNITHERM Connection"=w240) -> (w246:T25)
        n108 = Enqueue Element(queue=w252, element=w248, error in (no error)=w238) -> (error out=w251:errorcluster)  [unwired: 1 in, 2 out]
        n109 = Merge Errors(w239, w251) -> (w244:errorcluster)
      }
      frame "Clear Load" {
        # "Adjust the Impedance of the Unitherm."
        n110 = Unbundle By Name(w259) -> ("UNITHERM Connection"=w256:refnum<visa-resource-name>)
        n111 = call "FT10_Unitherm Clear Load.vi"("error in (no error)"=w254, "VISA Refnum in"=w256) -> ("error out"=w253:errorcluster, "VISA Refnum out"=w255:refnum<visa-resource-name>)  [unwired: 8 in]
        n112 = Bundle By Name(cluster=T28 {"Message"="", "Message Data"=variant} ("Message Cluster"), "Message"="Update Display", "Message Data"="Unitherm Load Cleared" ("L10n_Action 1 Pressed")) -> (w261:T28)
        n113 = Bundle By Name(cluster=w259, "UNITHERM Connection"=w255) -> (w260:T25)
        n114 = Enqueue Element(queue=w265, element=w261, error in (no error)=w254) -> (error out=w264:errorcluster)  [unwired: 1 in, 2 out]
        n115 = Merge Errors(w253, w264) -> (w258:errorcluster)
      }
      frame "Read Current" {
        # "0.0015 s at 130000000Hz"
        # "Adjust the Impedance of the Unitherm."
        n116 = Unbundle By Name(w283) -> ("M4X Connection"=w278:T26)
        n117 = call "FT10_M4X Single Capture with Autoscale.vi"("memsize"=194992, "Card Handle in"=w278) -> ("Data"=w274:waveform(sgl)[], "Card Handle out"=w279:u32)  [unwired: 8 in]
        n118 = Index Array(array=w274, index #1=0 ("index"), index #2=2 ("index")) -> (element #1=w268:waveform(sgl), element #2=w267:waveform(sgl))
        n119 = Multiply(x=w268, y=1000.0) -> (x*y=w271:waveform(dbl))
        n120 = Multiply(x=w267, y=10.0) -> (x*y=w270:waveform(dbl))
        n121 = Build Array(w271, w270) -> (w266:waveform(dbl)[])
        "Data" <- w266
        n122 = Bundle By Name(cluster=T28 {"Message"="", "Message Data"=variant} ("Message Cluster"), "Message"="Update Display", "Message Data"="\"Read Current\" pressed" ("L10n_Action 1 Pressed")) -> (w285:T28)
        n123 = for {
          tunnel: w266 -> [w290] mode=indexing
          tunnel: [w292] -> w269 mode=indexing
          tunnel: [w291] -> _ mode=indexing
          n124 = call "FT10_M4X Process Waveform.vi"("RF Waveform In"=w290) -> ("RF Waveform Out"=w291:waveform(sgl), "Measurements"=w292:T35)  [unwired: 12 in, 1 out]
        }
        "Array" <- w269
        n125 = Enqueue Element(queue=w289, element=w285, error in (no error)=w280) -> (error out=w288:errorcluster)  [unwired: 1 in, 2 out]
        n126 = Bundle By Name(cluster=w283, "M4X Connection"=w279) -> (w284:T25)
        n127 = Merge Errors(w288) -> (w282:errorcluster)
      }
      frame "7854 Set Config" {
        n128 = Variant To Data(type=T29 {"7854 Config Enum"=enum."Mono 1", "7854 Set Config"=FALSE}, Variant=w305) -> (data=w310:T29)  [unwired: 1 in, 1 out]
        n129 = Unbundle By Name(w310) -> ("7854 Config Enum"=w304:T10)
        n130 = Unbundle By Name(w308) -> ("PXI-7854R FPGA Reference"=w309:T27)
        n131 = call "FT10_FPGA_7854R Set Config.vi"("7854 Config Enum"=w304) -> ("Config string"=w295:string, "Conn2/DIO_8_15 In"=w302:bool[], "Conn2/DIO_0_7 In"=w303:bool[])  [unwired: 8 in]
        n132 = xnode "Read/Write Control"("FPGA VI Reference In"=w309, "Conn2/DIO_0_7 In"=w303, "Conn2/DIO_8_15 In"=w302) -> ("FPGA VI Reference Out"=w306:T27)  [unwired: 1 in, 1 out]
        n133 = Concatenate Strings("PXI-7854R Configuration Set to " ("Display Message"), w295) -> (w294:string)
        n134 = Bundle By Name(cluster=w308, "PXI-7854R FPGA Reference"=w306) -> (w307:T25)
        n135 = Bundle By Name(cluster=T28 {"Message"="", "Message Data"=variant} ("Message Cluster"), "Message"="Update Display", "Message Data"=w294) -> (w298:T28)
        n136 = Enqueue Element(queue=w293, element=w298, error in (no error)=w296) -> (error out=w297:errorcluster)  [unwired: 1 in, 2 out]
      }
      frame "Update Display" {
        # "Update Display - Convert the Message Data to a string to display in the Display Message indicator."
        n137 = Variant To Data(error in=w317, type="", Variant=w316) -> (data=→"Display Message":string, error out=w314:errorcluster)
      }
      frame "Exit" {
        w318 = bool[] [FALSE, FALSE, FALSE, FALSE, FALSE, FALSE, FALSE, FALSE] ("Conn2/DIO_0_7 In")
        # "Stop the VI."
        # "Release the message queue reference."
        # "Exit - Exit the application. Since this message was sent as a priority message (i.e., it was placed at the front of the queue), any cleanup code should run here, since the loop is about to stop. Any other messages in the queue will not be handled."
        n138 = Unbundle By Name(w326) -> ("UNITHERM Connection"=w328:refnum<visa-resource-name>, "PXI-7854R FPGA Reference"=w321:T27)
        n139 = xnode "Read/Write Control"("FPGA VI Reference In"=w321, "error in"=w322, "Conn2/DIO_0_7 In"=w318, "Conn2/DIO_8_15 In"=w318) -> ("FPGA VI Reference Out"=w319:T27, "error out"=w320:errorcluster)
        n140 = Release Queue(queue=w332, error in (no error)=w322) -> (error out=w330:errorcluster)  [unwired: 1 in, 2 out]
        n141 = call "FT10_Unitherm Clear Load.vi"("error in (no error)"=w322, "VISA Refnum in"=w328) -> ("error out"=w323:errorcluster, "VISA Refnum out"=w327:refnum<visa-resource-name>)  [unwired: 8 in]
        n142 = Bundle By Name(cluster=w326, "UNITHERM Connection"=w327, "PXI-7854R FPGA Reference"=w319) -> (w325:T25)
        n143 = Merge Errors(w323, w320, w330) -> (w324:errorcluster)
        n144 = local write "Display Message"("\"Stop\" button pressed" ("L10n_Stop Pressed")) -> ()
      }
      frame Default {
        # "The Default case only runs if there is a message that isn't defined in any of the other cases. Generate an error if this occurs."
        n145 = xnode "Error Ring"("parameter 0"=w336) -> ("error out"=w334:errorcluster)
        n146 = call <vilib>:"Simple Error Handler.vi"("error in (no error)"=w334) -> ()  [unwired: 4 in, 5 out]
      }
    }
  }
  n147 = while {
    tunnel: w2 -> [w346]
    tunnel: [w344] -> w14
    stop <- w345 stop-if-true
    # "Event Handling Loop"
    n148 = event shown="[0] \"Fornax Action 1\": Value Change" {
      selector: _ -> [_ _ _ _ _ _ _ _ _ _ _ _]
      dyn-events: _ -> [_ _ _ _ _ _ _ _ _ _ _ _]
      timeout: _ -> [_ _ _ _ _ _ _ _ _ _ _ _]
      tunnel: [_ _ _ _ _ _ _ _ _ _ TRUE TRUE] -> w345
      tunnel: w346 -> [w349 w363 w370 w379 w391 w397 w412 w430 w436 w438 w456 w460]
      tunnel: [w348 w362 w369 w378 w390 w398 w411 w429 w435 w440 w459 w463] -> w344
      event "Fornax Action 1": Value Change {
        # "Enqueue an \"Action 1\" message."
        n149 = event-data() -> ()  [unwired: 1 in, 1 out]
        n150 = Enqueue Element(queue=w349, element=T28 {"Message"="Fornax Action 1", "Message Data"=variant}) -> (error out=w348:errorcluster)  [unwired: 2 in, 2 out]
      }
      event Value Change {
        # "When \"Fornax Set Monopolar Command\" button is held down command will continuously execute. Once button is no longer being held. Command turns false and stops."
        n151 = event-data() -> ()  [unwired: 1 in, 1 out]
        n152 = Bundle By Name(cluster=T34 {"Serial Number"="CAMM_INTERNAL_GENERIC", "EnergyChannelID"=enum."EC_MONO_1", "CutMode"=enum."SPRAY_MODE", "CoagMode"=enum."SPRAY_MODE", "CutPowerCommand"=enum."POWER_NO_CHANGE", "CoagPowerCommand"=enum."POWER_NO_CHANGE", "Fornax Set Monopolar Command"=FALSE}, "Serial Number"="Serial Number", "EnergyChannelID"="EnergyChannelID", "CutMode"="CutMode", "CoagMode"="CoagMode", "CutPowerCommand"="CutPowerCommand", "CoagPowerCommand"="CoagPowerCommand", "Fornax Set Monopolar Command"="Fornax Set Monopolar Command") -> (w350:T34)
        n153 = Bundle By Name(cluster=T28 {"Message"="Fornax Connect/Disconnect", "Message Data"=variant} ("element"), "Message"="Fornax Set Monopolar Command", "Message Data"=w350) -> (w359:T28)
        n154 = Enqueue Element(queue=w363, element=w359) -> (error out=w362:errorcluster)  [unwired: 2 in, 2 out]
      }
      event Value Change {
        # "Enqueue an \"Action 1\" message."
        n155 = event-data() -> ()  [unwired: 1 in, 1 out]
        n156 = case shown="True" "Fornax Connect/Disconnect" {
          tunnel: ["Connect" ("Boolean Text.Text") "Disconnect" ("Boolean Text.Text")] -> w364
          frame False {
          }
          frame True {
          }
        }
        n157 = property on="Fornax Connect/Disconnect" class="Bool (strict)"("BoolText.Text"=w364) -> ()  [unwired: 2 in, 2 out]
        n158 = Bundle By Name(cluster=T28 {"Message"="Fornax Connect/Disconnect", "Message Data"=variant} ("element"), "Message"="Fornax Connect/Disconnect", "Message Data"="Fornax Connect/Disconnect") -> (w366:T28)
        n159 = Enqueue Element(queue=w370, element=w366) -> (error out=w369:errorcluster)  [unwired: 2 in, 2 out]
      }
      event Value Change {
        # "Enqueue an \"Action 1\" message."
        n160 = event-data() -> ()  [unwired: 1 in, 1 out]
        n161 = case shown="True" "M4X Connect/Disconnect" {
          tunnel: ["Connect" ("Boolean Text.Text") "Disconnect" ("Boolean Text.Text")] -> w373
          frame False {
          }
          frame True {
          }
        }
        n162 = property on="M4X Connect/Disconnect" class="Bool (strict)"("BoolText.Text"=w373) -> ()  [unwired: 2 in, 2 out]
        n163 = Bundle By Name(cluster=T28 {"Message"="Fornax Connect/Disconnect", "Message Data"=variant} ("element"), "Message"="M4X Connect/Disconnect", "Message Data"="M4X Connect/Disconnect") -> (w375:T28)
        n164 = Enqueue Element(queue=w379, element=w375) -> (error out=w378:errorcluster)  [unwired: 2 in, 2 out]
      }
      event Value Change {
        # "Enqueue an \"Action 1\" message."
        n165 = event-data() -> ()  [unwired: 1 in, 1 out]
        n166 = Bundle By Name(cluster=T31 {"Unitherm Connect/Disconnect"=FALSE, "Unitherm Refnum in"=""}, "Unitherm Connect/Disconnect"="Unitherm Connect/Disconnect", "Unitherm Refnum in"="Unitherm Refnum in") -> (w386:T31)
        n167 = case shown="True" "Unitherm Connect/Disconnect" {
          tunnel: ["Connect" ("Boolean Text.Text") "Disconnect" ("Boolean Text.Text")] -> w382
          frame False {
          }
          frame True {
          }
        }
        n168 = property on="Unitherm Connect/Disconnect" class="Bool (strict)"("BoolText.Text"=w382) -> ()  [unwired: 2 in, 2 out]
        n169 = Bundle By Name(cluster=T28 {"Message"="Fornax Connect/Disconnect", "Message Data"=variant} ("element"), "Message"="Unitherm Connect/Disconnect", "Message Data"=w386) -> (w387:T28)
        n170 = Enqueue Element(queue=w391, element=w387) -> (error out=w390:errorcluster)  [unwired: 2 in, 2 out]
      }
      event Value Change {
        n171 = event-data() -> ()  [unwired: 1 in, 1 out]
        n172 = case shown="True" "7854 Connect/Disconnect" {
          tunnel: ["Connect" ("Boolean Text.Text") "Disconnect" ("Boolean Text.Text")] -> w395
          frame False {
          }
          frame True {
          }
        }
        n173 = Bundle By Name(cluster=T32 {"PXI-7854R Resource"="PXI1Slot6", "75kHz"=TRUE, "uSec Off"=6, "uSec On"=7, "7854 Connect/Disconnect"=FALSE}, "7854 Connect/Disconnect"="7854 Connect/Disconnect", "75kHz"="75kHz", "uSec Off"="uSec Off", "uSec On"="uSec On", "PXI-7854R Resource"="resource name") -> (w399:T32)
        n174 = property on="7854 Connect/Disconnect" class="Bool (strict)"("BoolText.Text"=w395) -> ()  [unwired: 2 in, 2 out]
        n175 = Bundle By Name(cluster=T28 {"Message"="Fornax Connect/Disconnect", "Message Data"=variant} ("element"), "Message"="7854 Connect/Disconnect", "Message Data"=w399) -> (w405:T28)
        n176 = Enqueue Element(queue=w397, element=w405) -> (error out=w398:errorcluster)  [unwired: 2 in, 2 out]
      }
      event Value Change {
        # "Enqueue an \"Action 1\" message."
        n177 = event-data() -> ()  [unwired: 1 in, 1 out]
        n178 = disable-structure shown="Disabled" {
          frame Disabled {
            n179 = call "FT10_Unitherm Ask Dialog - Set Load.vi"() -> ()  [unwired: 11 in, 1 out]
          }
          frame Enabled {
          }
        }
        n180 = case shown="True" "Set Load" {
          tunnel: w412 -> [w418 w424]
          tunnel: [w414 w420] -> w411
          tunnel: "Load (Ohms)" -> [w413 _]
          frame True {
            n181 = Bundle By Name(cluster=T28 {"Message"="Fornax Connect/Disconnect", "Message Data"=variant} ("element"), "Message"="Set Load", "Message Data"=w413) -> (w415:T28)
            n182 = Enqueue Element(queue=w418, element=w415) -> (error out=w414:errorcluster)  [unwired: 2 in, 2 out]
          }
          frame False {
            n183 = Bundle By Name(cluster=T28 {"Message"="Fornax Connect/Disconnect", "Message Data"=variant} ("element"), "Message"="Update Display", "Message Data"="Unitherm Set Load Canceled" ("Message")) -> (w421:T28)
            n184 = Enqueue Element(queue=w424, element=w421) -> (error out=w420:errorcluster)  [unwired: 2 in, 2 out]
          }
        }
      }
      event Value Change {
        # "Enqueue an \"Action 1\" message."
        n185 = event-data() -> ()  [unwired: 1 in, 1 out]
        n186 = Bundle By Name(cluster=T28 {"Message"="Fornax Connect/Disconnect", "Message Data"=variant} ("element"), "Message"="Clear Load", "Message Data"="Clear Load") -> (w426:T28)
        n187 = Enqueue Element(queue=w430, element=w426) -> (error out=w429:errorcluster)  [unwired: 2 in, 2 out]
      }
      event Value Change {
        # "Enqueue an \"Action 1\" message."
        n188 = event-data() -> ()  [unwired: 1 in, 1 out]
        n189 = Bundle By Name(cluster=T28 {"Message"="Fornax Connect/Disconnect", "Message Data"=variant} ("element"), "Message"="Read Current", "Message Data"="Read Current") -> (w432:T28)
        n190 = Enqueue Element(queue=w436, element=w432) -> (error out=w435:errorcluster)  [unwired: 2 in, 2 out]
      }
      event Value Change {
        n191 = event-data() -> ()  [unwired: 1 in, 1 out]
        n192 = disable-structure shown="Disabled" {
          frame Disabled {
            n193 = call "FT10_FPGA_7854R Ask Dialog - Set Config.vi"() -> ()  [unwired: 11 in, 1 out]
          }
          frame Enabled {
          }
        }
        n194 = case shown="True" "7854 Set Config" {
          selector: "7854 Set Config" -> [_ w448]
          tunnel: [w441 w450] -> w440
          tunnel: "7854 Config Enum" -> [_ w449]
          tunnel: w438 -> [w442 w447]
          frame False {
            n195 = Bundle By Name(cluster=T28 {"Message"="Fornax Connect/Disconnect", "Message Data"=variant} ("element"), "Message"="Update Display", "Message Data"="PXI-7854R Set Configuration Canceled" ("Message")) -> (w446:T28)
            n196 = Enqueue Element(queue=w442, element=w446) -> (error out=w441:errorcluster)  [unwired: 2 in, 2 out]
          }
          frame True {
            n197 = Bundle By Name(cluster=T29 {"7854 Config Enum"=enum."Mono 1", "7854 Set Config"=FALSE}, "7854 Config Enum"=w449, "7854 Set Config"=w448) -> (w451:T29)
            n198 = Bundle By Name(cluster=T28 {"Message"="Fornax Connect/Disconnect", "Message Data"=variant} ("element"), "Message"="7854 Set Config", "Message Data"=w451) -> (w454:T28)
            n199 = Enqueue Element(queue=w447, element=w454) -> (error out=w450:errorcluster)  [unwired: 2 in, 2 out]
          }
        }
      }
      event Value Change {
        # "Stop the VI."
        # "Enqueue an \"Exit\" message. Note that the Enqueue Element At Opposite End function is used to place this priority \"Exit\" message at the front of the queue ahead of all other messages."
        n200 = event-data() -> ()  [unwired: 1 in, 1 out]
        n201 = Enqueue Element At Opposite End(queue=w456, element=T28 {"Message"="Exit", "Message Data"=variant}) -> (error out=w459:errorcluster)  [unwired: 2 in, 2 out]
      }
      event Panel Close? {
        # "Stop the VI."
        # "Enqueue an \"Exit\" message. Note that the Enqueue Element At Opposite End function is used to place this priority \"Exit\" message at the front of the queue ahead of all other messages."
        n202 = event-data() -> ()  [unwired: 1 in, 1 out]
        n203 = Enqueue Element At Opposite End(queue=w460, element=T28 {"Message"="Exit", "Message Data"=variant}) -> (error out=w463:errorcluster)  [unwired: 2 in, 2 out]
        n204 = event-data() -> ()  [unwired: 2 in, 1 out]
      }
    }
  }
  n205 = Merge Errors(w14, w15) -> (w8:errorcluster)
  n206 = call <vilib>:"Simple Error Handler.vi"("error in (no error)"=w8) -> ()  [unwired: 4 in, 5 out]
